vi "drop_sample.vi"(10 "trigger in":bool[](array[boolean])=[FALSE, FALSE, FALSE, FALSE, FALSE, FALSE, FALSE, FALSE]) -> (2 "drop sample":bool[](array[boolean]))   [LabVIEW 2012]
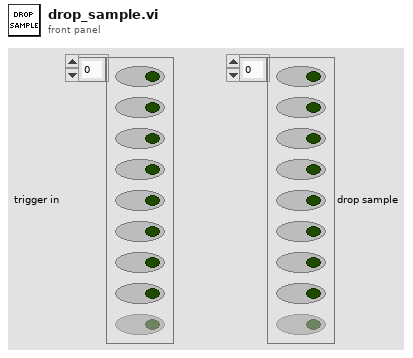
[diagram p1: front panel]
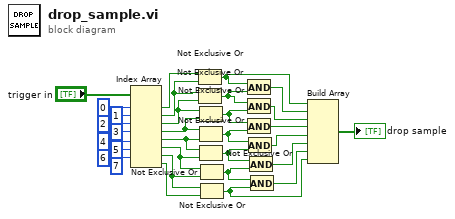
[diagram p0: block diagram]
diagram:
  (unwired) 7 ("index")
  n1 = Index Array(array="trigger in", index #1=0 ("index"), index #2=1 ("index"), index #3=2 ("index"), index #4=3 ("index"), index #5=4 ("index"), index #6=5 ("index"), index #7=6 ("index")) -> (element #1=w22:bool, element #2=w21:bool, element #3=w20:bool, element #4=w19:bool, element #5=w18:bool, element #6=w17:bool, element #7=w16:bool, element #8=w15:bool)  [unwired: 1 in]
  n2 = Not Exclusive Or(1:w21, 2:w22) -> (0:w9:bool)
  n3 = Not Exclusive Or(1:w20, 2:w21) -> (0:w14:bool)
  n4 = Not Exclusive Or(1:w19, 2:w20) -> (0:w13:bool)
  n5 = Not Exclusive Or(1:w18, 2:w19) -> (0:w12:bool)
  n6 = Not Exclusive Or(1:w17, 2:w18) -> (0:w11:bool)
  n7 = Not Exclusive Or(1:w16, 2:w17) -> (0:w10:bool)
  n8 = Not Exclusive Or(1:w15, 2:w16) -> (0:w8:bool)
  n9 = And(x=w9, y=w14) -> (x .and. y?=w6:bool)
  n10 = And(x=w14, y=w13) -> (x .and. y?=w5:bool)
  n11 = And(x=w13, y=w12) -> (x .and. y?=w2:bool)
  n12 = And(x=w12, y=w11) -> (x .and. y?=w3:bool)
  n13 = And(x=w11, y=w10) -> (x .and. y?=w4:bool)
  n14 = And(x=w10, y=w8) -> (x .and. y?=w7:bool)
  n15 = Build Array(w9, w6, w5, w2, w3, w4, w7, w8) -> (→"drop sample":bool[])
